vi "Update Status.vi"(8 "error in (no error)":errorcluster, 9 "Serial Number":string, 10 "Sensor Status":i32, 11 "ImageHandler in":refnum<class "ImageHandler.lvclass">) -> (0 "error out":errorcluster, 3 "ImageHandler out":refnum<class "ImageHandler.lvclass">)   [LabVIEW 2021, in "ImageHandler.lvlib" / "ImageHandler.lvclass"]
uses:
  ImageHandler.lvclass
  C:/Program Files/National Instruments/LabVIEW 2021/vi.lib/ActorFramework/Actor/Actor.lvclass
  <vilib>/ActorFramework/Actor/Actor.lvclass/Actor.ctl
  ImageHandler - Controller -- Interface/ImageHandler - Controller -- Interface Messages/Connection Status Msg/Connection Status Msg.lvclass/Connection Status Msg.ctl
  <vilib>/ActorFramework/Message Enqueuer/Message Enqueuer.lvclass/Message Enqueuer.ctl
  <vilib>/ActorFramework/Message Enqueuer/Enqueue.vi
  ImageHandler - Controller -- Interface/ImageHandler - Controller -- Interface Messages/Connection Status Msg/Connection Status Msg.lvclass
  C:/Program Files/National Instruments/LabVIEW 2021/vi.lib/ActorFramework/Message/Message.lvclass
  <vilib>/ActorFramework/Message Priority Queue/Priority Enqueue.vi
  <vilib>/ActorFramework/Actor/Actor.lvclass
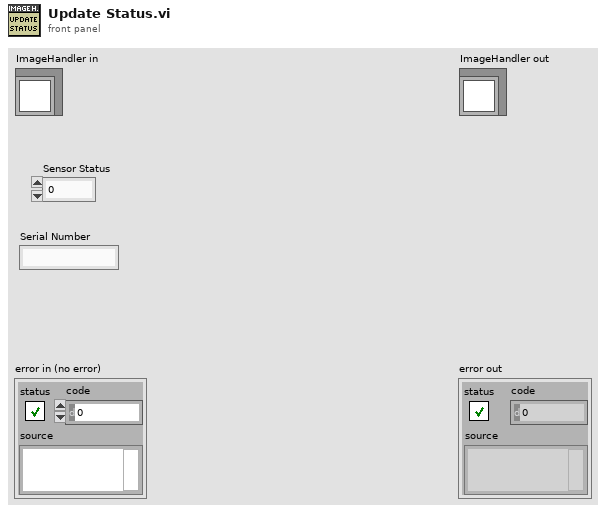
[diagram p1: front panel]
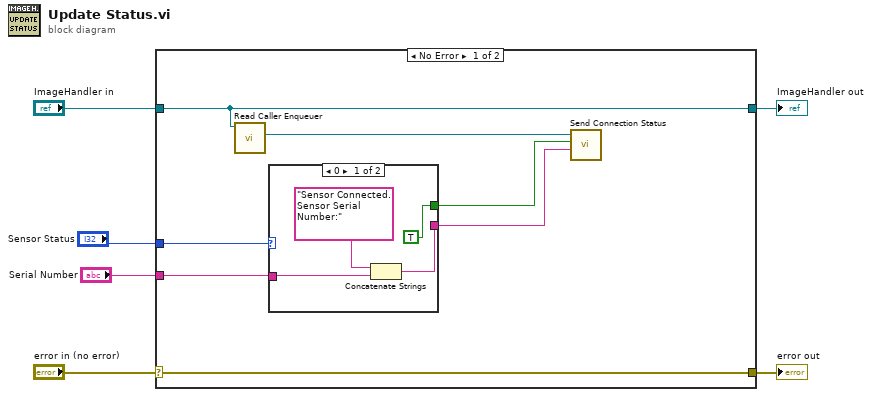
[diagram p0: block diagram]
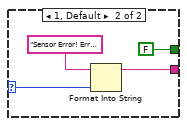
[diagram p2: hidden frame]
diagram:
  n1 = case shown="No Error" "error in (no error)" {
    selector: "error in (no error)" -> [w13 w23]
    tunnel: [w13 w23] -> w5
    tunnel: [w8 w22] -> w3
    tunnel: "ImageHandler in" -> [w8 w22]
    tunnel: "Sensor Status" -> [w10 _]
    tunnel: "Serial Number" -> [w9 _]
    frame No Error {
      n2 = call <vilib>:"Read Caller Enqueuer.vi"("Actor"=w8) -> ("Caller Enqueuer"=w7:refnum<class "Message Enqueuer.lvclass">)  [unwired: 10 in]
      n3 = case shown="0" w10 {
        selector: w10 -> [_ w20]
        tunnel: [TRUE FALSE] -> w11
        tunnel: w9 -> [w15 _]
        tunnel: [w14 w18] -> w12
        frame 0 {
          n4 = Concatenate Strings("Sensor Connected. Sensor Serial Number:", w15) -> (w14:string)
        }
        frame 1, Default {
          n5 = Format Into String(initial string="Sensor Error! Error Code:", w20) -> (resulting string=w18:string)  [unwired: 2 in, 1 out]
        }
      }
      n6 = call "Send Connection Status.vi"("Remarks"=w12, "Status"=w11, "Message Enqueuer"=w7) -> ()  [unwired: 7 in, 2 out]
    }
    frame Error {
    }
  }
  "error out" <- w5
  "ImageHandler out" <- w3
